vi "Purchase And Dispensing.vi"(7 "Products":T1, 8 "error in (no error)":errorcluster, 9 "Currency in":T3, 10 "Product_Data":T2[](array[typedef]), 11 "Data in":T5) -> (0 "error out":errorcluster, 1 "Currency out":T3, 2 "Product_Data out":T2[](array[typedef]), 3 "Data out":T5)   [LabVIEW 2026]
uses:
  controls/Product.ctl
  controls/Currency.ctl
  controls/Currency Enum.ctl
  controls/Data.ctl
  controls/Products Enum.ctl
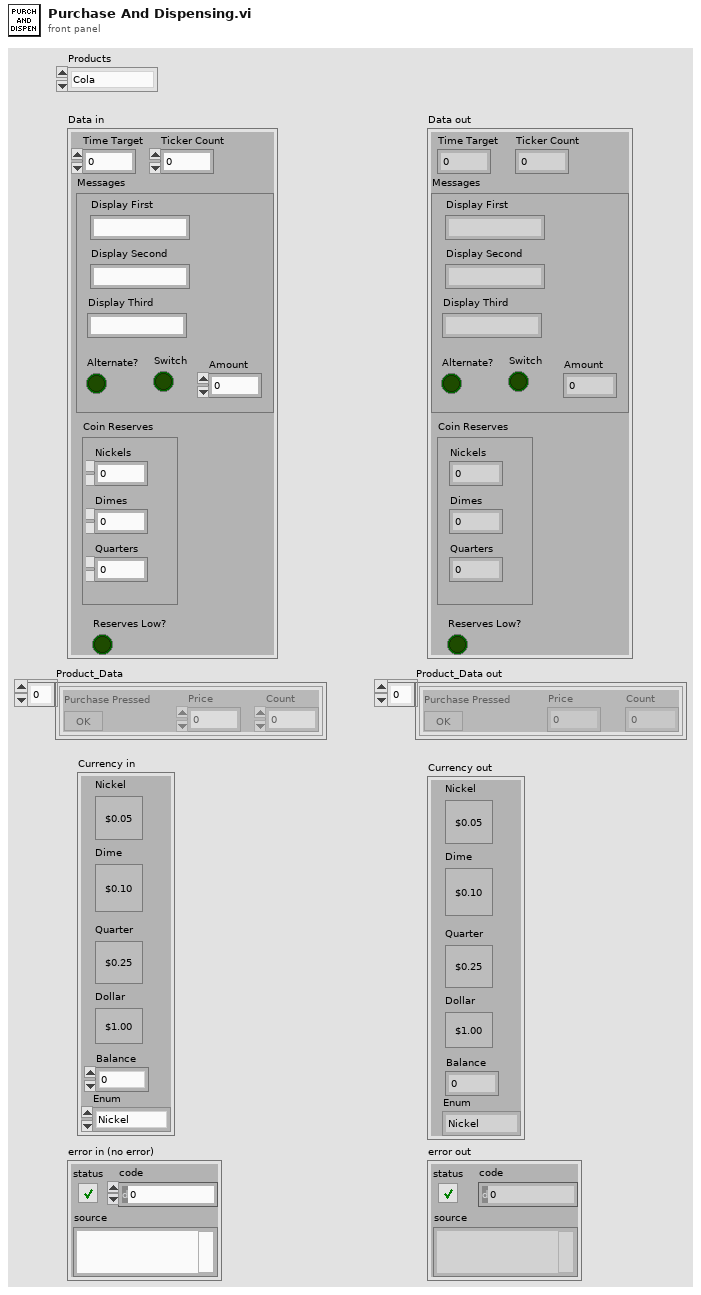
[diagram p1: front panel]
types:
  T1 = typedef "Products Enum.ctl" = enum16{"Cola", "Chips", "Candy"}
  T2 = typedef "Product.ctl" = cluster{"Purchase Pressed":bool, "Price":dbl, "Count":i32}
  T3 = typedef "Currency.ctl" = cluster{"Nickel":bool, "Dime":bool, "Quarter":bool, "Dollar":bool, "Balance":dbl, "Enum":T4}
  T4 = typedef "Currency Enum.ctl" = enum16{"Nickel", "Dime", "Quarter", "Dollar"}
  T5 = typedef "Data.ctl" = cluster{"Time Target":dbl, "Messages":cluster{"Display First":string, "Display Second":string, "Alternate?":bool, "Switch":bool, "Display Third":string, "Amount":i32}, "Ticker Count":dbl, "Coin Reserves":cluster{"Nickels":i32, "Dimes":i32, "Quarters":i32}, "Reserves Low?":bool}
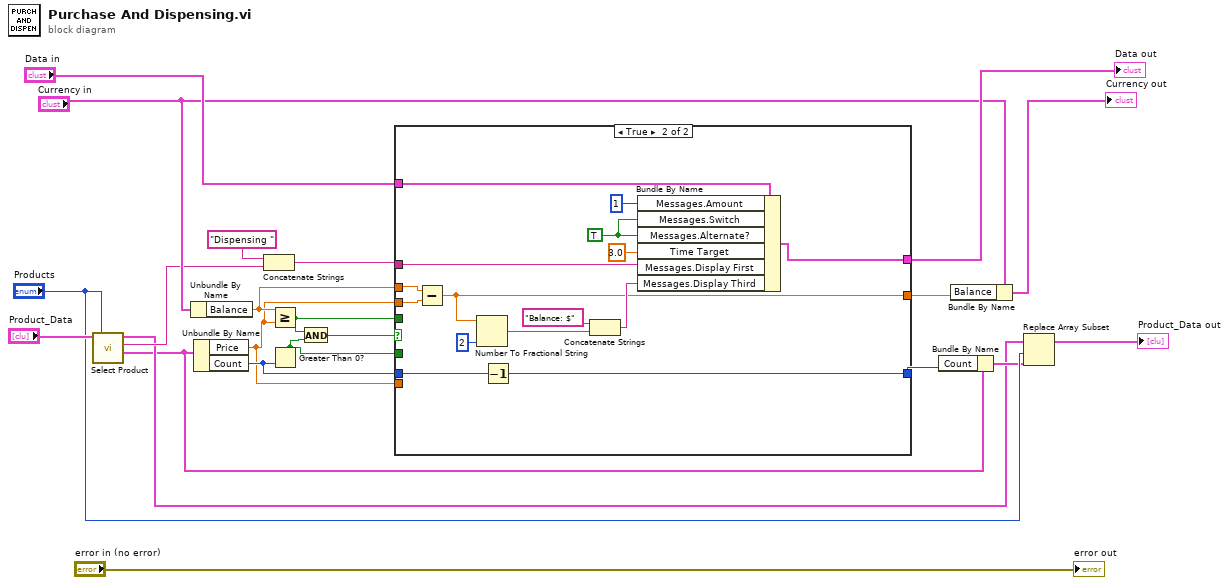
[diagram p0: block diagram]
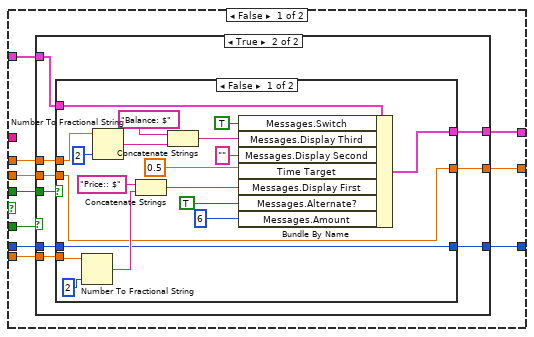
[diagram p2: hidden frame]
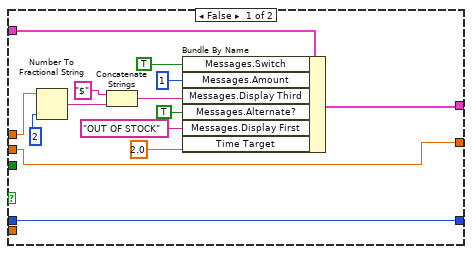
[diagram p3: hidden frame]
diagram:
  n1 = call "Select Product.vi"("Products in"="Products", "Product_Data in"="Product_Data") -> ("Product"=w1:T2, "String"=w5:string, "Product_Data out"=w2:T2[])  [unwired: 6 in, 1 out]
  n2 = Unbundle By Name("Currency in") -> ("Balance"=w17:dbl)
  n3 = Unbundle By Name(w1) -> ("Price"=w10:dbl, "Count"=w15:i32)
  n4 = Concatenate Strings("Dispensing ", w5) -> (w7:string)
  n5 = Greater Or Equal?(x=w17, y=w10) -> (x >= y?=w11:bool)
  n6 = Greater Than 0?(x=w15) -> (x > 0?=w12:bool)
  n7 = And(x=w11, y=w12) -> (x .and. y?=w14:bool)
  n8 = case shown="True" w14 {
    tunnel: w15 -> [w27 w87]
    tunnel: [w26 w86] -> w16
    tunnel: w17 -> [w28 w92]
    tunnel: w10 -> [w25 w91]
    tunnel: [w24 w79] -> w19
    tunnel: "Data in" -> [w23 w90]
    tunnel: w7 -> [_ w89]
    tunnel: [w29 w78] -> w21
    tunnel: w12 -> [w32 _]
    tunnel: w11 -> [w31 _]
    tunnel: w10 -> [w30 _]
    frame False {
      n9 = case shown="True" w32 {
        tunnel: w31 -> [_ w55]
        tunnel: w30 -> [_ w53]
        tunnel: [w44 w52] -> w29
        tunnel: w28 -> [w37 w51]
        tunnel: w27 -> [w43 w50]
        tunnel: [w43 w49] -> w26
        tunnel: w25 -> [w42 w48]
        tunnel: [w42 w47] -> w24
        tunnel: w23 -> [w34 w54]
        frame False {
          n10 = Number To Fractional String(number=w37, precision (6)=i16 2) -> (F-format string=w39:string)  [unwired: 2 in]
          n11 = Concatenate Strings("$", w39) -> (w38:string)
          n12 = Bundle By Name(cluster=w34, "Messages.Switch"=TRUE, "Messages.Amount"=1, "Messages.Display Third"=w38, "Messages.Alternate?"=TRUE, "Messages.Display First"="OUT OF STOCK", "Time Target"=2.0) -> (w44:T5)
        }
        frame True {
          n13 = case shown="False" w55 {
            tunnel: w54 -> [w74 w77]
            tunnel: w53 -> [w71 _]
            tunnel: [w68 w77] -> w52
            tunnel: w51 -> [w66 _]
            tunnel: w50 -> [w63 w75]
            tunnel: [w63 w75] -> w49
            tunnel: w48 -> [w62 w76]
            tunnel: [w62 w76] -> w47
            frame False {
              n14 = Number To Fractional String(number=w71, precision (6)=i16 2) -> (F-format string=w70:string)  [unwired: 2 in]
              n15 = Number To Fractional String(number=w66, precision (6)=i16 2) -> (F-format string=w64:string)  [unwired: 2 in]
              n16 = Concatenate Strings("Price:: $", w70) -> (w69:string)
              n17 = Concatenate Strings("Balance: $", w64) -> (w60:string)
              n18 = Bundle By Name(cluster=w74, "Messages.Switch"=TRUE, "Messages.Display Third"=w60, "Messages.Display Second"="", "Time Target"=0.5, "Messages.Display First"=w69, "Messages.Alternate?"=TRUE, "Messages.Amount"=6) -> (w68:T5)
            }
            frame True {
            }
          }
        }
      }
    }
    frame True {
      w80 = TRUE ("Messages.Alternate?")
      n19 = Subtract(x=w92, y=w91) -> (x-y=w79:dbl)
      n20 = Number To Fractional String(number=w79, precision (6)=i16 2) -> (F-format string=w83:string)  [unwired: 2 in]
      n21 = Decrement(x=w87) -> (x-1=w86:i32)
      n22 = Concatenate Strings("Balance: $", w83) -> (w81:string)
      n23 = Bundle By Name(cluster=w90, "Messages.Amount"=1, "Messages.Switch"=w80, "Messages.Alternate?"=w80, "Time Target"=3.0, "Messages.Display First"=w89, "Messages.Display Third"=w81) -> (w78:T5)
    }
  }
  "Data out" <- w21
  n24 = Bundle By Name(cluster=w1, "Count"=w16) -> (w3:T2)
  n25 = Bundle By Name(cluster="Currency in", "Balance"=w19) -> (→"Currency out":T3)
  n26 = Replace Array Subset(array=w2, new element=w3, index="Products") -> (→"Product_Data out":T2[])
  "error out" <- "error in (no error)"
